vi "lee digitales.vi"(0 "nº equip":u8, 1 "COM DATA":T1) -> (2 "error out":errorcluster, 3 "logicas":string, 4 "COM FAIL":bool)   [LabVIEW 2010]
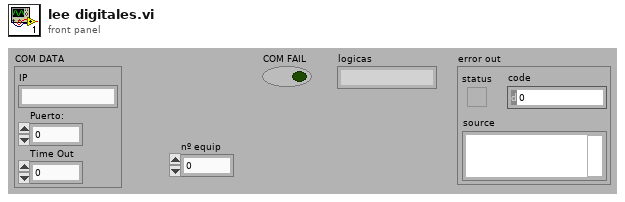
[diagram p1: front panel]
types:
  T1 = cluster{"IP ":string, "Puerto:":u16, "Time Out":u16}
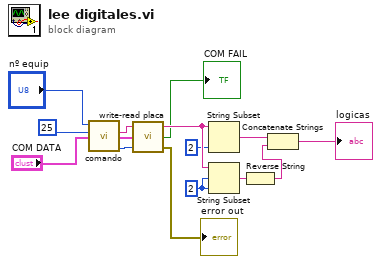
[diagram p0: block diagram]
diagram:
  w9 = 2 ("length (rest)")
  n1 = call "comando.vi"("Comando:"=u8 25, "Equipo Nº"="nº equip") -> ("Bytes OUT"=w3:u16, "comando"=w2:string)  [unwired: 5 in]
  n2 = call "write-read placa.vi"("Write Command"=w2, "COM DATA"="COM DATA", "bytes"=w3) -> ("LECTURA"=w10:string, "COM FAIL"=→"COM FAIL":bool, "error out"=→"error out":errorcluster)  [unwired: 2 in]
  n3 = String Subset(string=w10, length (rest)=2 ("length (rest)")) -> (substring=w12:string)  [unwired: 1 in]
  n4 = String Subset(string=w10, offset (0)=w9, length (rest)=w9) -> (substring=w11:string)
  n5 = Reverse String(1:w11) -> (0:w14:string)
  n6 = Concatenate Strings(w12, w14) -> (→"logicas":string)
